vi "Read Display Metadata.vi"(8 "error in":errorcluster, 11 "Value in":refnum<class "Value.lvclass">) -> (0 "error out":errorcluster, 1 "has display metadata?":bool, 2 "display metadata":T1, 3 "Value out":refnum<class "Value.lvclass">)   [LabVIEW 2020, in "Value.lvlib" / "Value.lvclass"]
uses:
  Value.lvclass
  Display Metadata.ctl
  Value.lvlib
  <vilib>/addons/Tools/Unicode/UTF8 Tools.lvlib
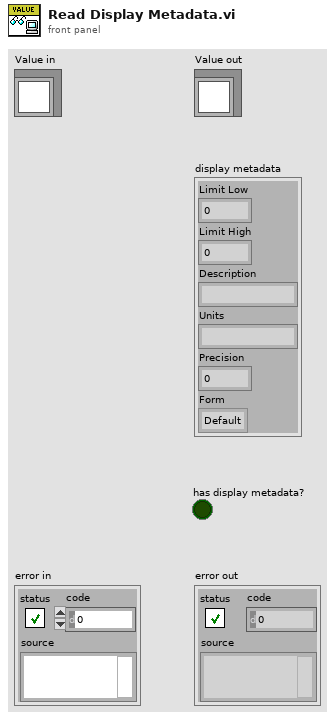
[diagram p1: front panel]
types:
  T1 = typedef "Value.lvlib/Display Metadata.ctl" = cluster{"Limit Low":dbl, "Limit High":dbl, "Description":string, "Units":string, "Precision":i32, "Form":enum32{"Default", "String", "Binary", "Decimal", "Hex", "Exponential", "Engineering"}}
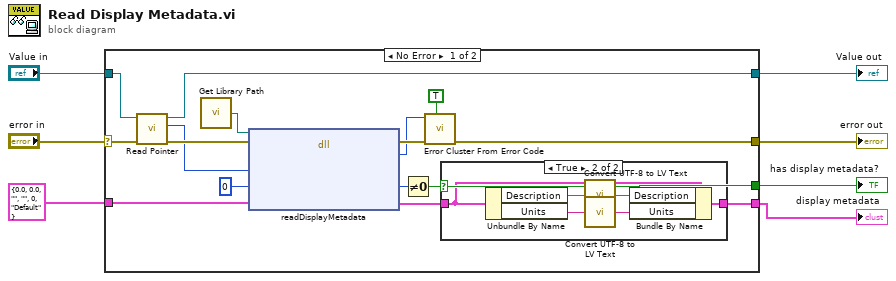
[diagram p0: block diagram]
diagram:
  n1 = case shown="No Error" "error in" {
    selector: "error in" -> [w18 w32]
    tunnel: [w19 w32] -> w7
    tunnel: "Value in" -> [w16 w31]
    tunnel: [w14 w31] -> w4
    tunnel: T1 {"Limit Low"=0.0, "Limit High"=0.0, "Description"="", "Units"="", "Precision"=0, "Form"=enum."Default"} ("Display") -> [w13 _]
    tunnel: [w10 _] -> w2
    tunnel: [w8 _] -> w1
    frame No Error {
      n2 = call-dynamic "Read Pointer.vi"("error in (no error)"=w18, "Value in"=w16) -> ("error out"=w17:errorcluster, "pointer"=w15:i64, "Value out"=w14:refnum<class "Value.lvclass">)  [unwired: 7 in]
      n3 = call "Get Library Path.vi"() -> ("Path"=w23:path)  [unwired: 1 in]
      n4 = dll-call lib="?" fn="readDisplayMetadata"(path in=w23, error in=w17, "value"=w15, "has display metadata?"=i16 0, "display metadata"=w13) -> (error out=w21:errorcluster, "err_code"=w20:i32, "has display metadata?"=w12:i16, "display metadata"=w9:T1)  [unwired: 2 in, 1 out]
      n5 = Not Equal To 0?(x=w12) -> (x != 0?=w10:bool)
      n6 = call <vilib>:"Error Cluster From Error Code.vi"("show call chain? (False)"=TRUE, "error in (no error)"=w21, "error code (0)"=w20) -> ("error out"=w19:errorcluster)  [unwired: 6 in]
      n7 = case shown="True" w10 {
        tunnel: w9 -> [w24 w28]
        tunnel: [w24 w25] -> w8
        frame False {
        }
        frame True {
          n8 = Unbundle By Name(w28) -> ("Description"=w30:string, "Units"=w29:string)
          n9 = call <vilib>:"Convert UTF-8 to LV Text.vi"("UTF-8 Text"=w30) -> ("LV Text"=w27:string)  [unwired: 13 in, 1 out]
          n10 = call <vilib>:"Convert UTF-8 to LV Text.vi"("UTF-8 Text"=w29) -> ("LV Text"=w26:string)  [unwired: 13 in, 1 out]
          n11 = Bundle By Name(cluster=w28, "Description"=w27, "Units"=w26) -> (w25:T1)
        }
      }
    }
    frame Error {
    }
  }
  "error out" <- w7
  "Value out" <- w4
  "has display metadata?" <- w2
  "display metadata" <- w1
